vi "Configure Simultaneous Measurement.vi"(6 "Enable Voltage Measurement (False)":bool, 7 "Enable Current Measurement (False)":bool, 8 "error in (no error)":errorcluster {"code" format="%.0x"}, 10 "Channel Name (1)":string="1", 11 "VISA resource name":refnum<visa-resource-name>) -> (0 "error out":errorcluster {"code" format="%.0x"}, 3 "VISA resource name out":refnum<visa-resource-name>)   [LabVIEW 2018, in "Agilent N6700 Series.lvlib"]
doc: "Configures simultaneous voltage and current measurement."
uses:
  Agilent N6700 Series.lvlib
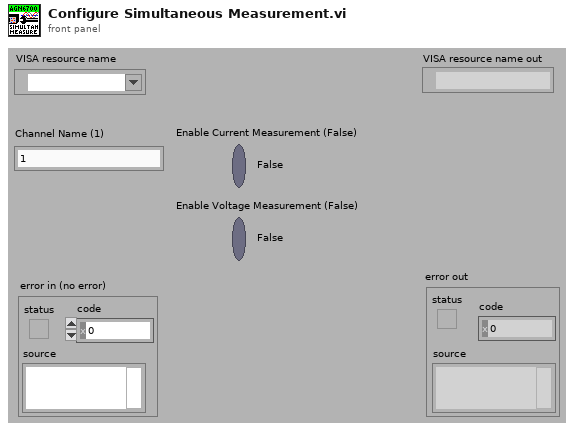
[diagram p1: front panel]
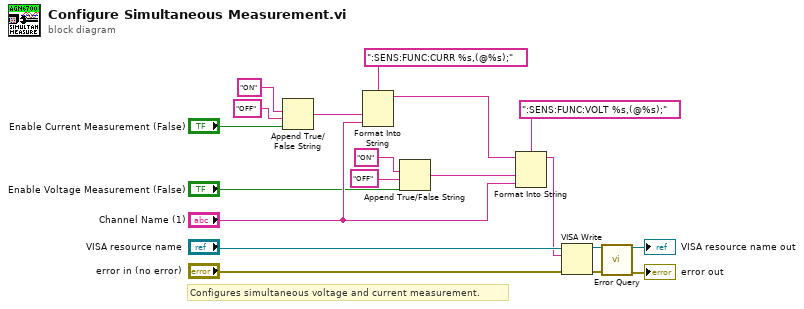
[diagram p0: block diagram]
diagram:
  # "Configures simultaneous voltage and current measurement."
  n1 = Append True/False String(1:"Enable Current Measurement (False)", 2:"OFF", 3:"ON") -> (0:w8:string)  [unwired: 1 in]
  n2 = Format Into String(format string=":SENS:FUNC:CURR %s,(@%s);", w8, "Channel Name (1)") -> (resulting string=w7:string)  [unwired: 2 in, 1 out]
  n3 = Append True/False String(1:"Enable Voltage Measurement (False)", 2:"OFF", 3:"ON") -> (0:w3:string)  [unwired: 1 in]
  n4 = Format Into String(format string=":SENS:FUNC:VOLT %s,(@%s);", initial string=w7, w3, "Channel Name (1)") -> (resulting string=w12:string)  [unwired: 1 in, 1 out]
  n5 = VISA Write(VISA resource name="VISA resource name", write buffer=w12, error in (no error)="error in (no error)") -> (VISA resource name out=w15:refnum<visa-resource-name>, error out=w14:errorcluster)  [unwired: 1 out]
  n6 = call "Error Query.vi"("VISA resource name"=w15, "error in (no error)"=w14) -> ("VISA resource name out"=→"VISA resource name out":refnum<visa-resource-name>, "error out"=→"error out":errorcluster)  [unwired: 10 in, 2 out]
